vi "celiang.vi"(7 "error in":errorcluster) -> (27 "error out":errorcluster)   [LabVIEW 2014]
uses:
  <vilib>/vision/Image Controls.llb/Vision Info Type2.ctl
  <vilib>/vision/Pattern Matching.llb/IMAQ Curve Parameters.ctl
  <vilib>/vision/NI_Vision_Development_Module.lvlib
panel:
  out "Image Out":T1(plugin-control)
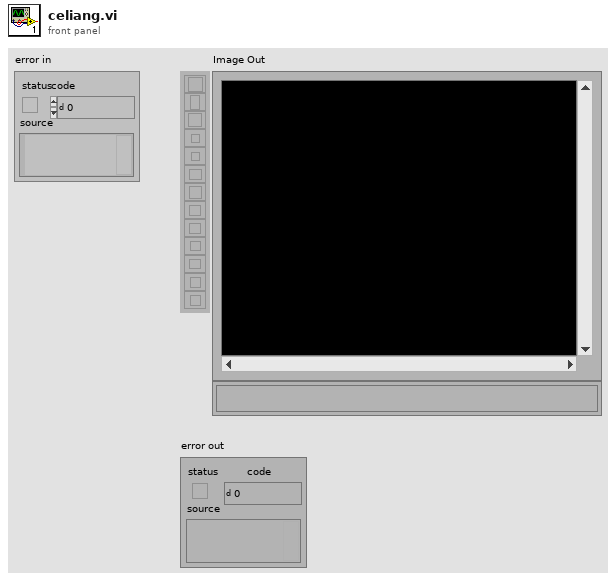
[diagram p1: front panel]
types:
  T1 = typedef "IMAQ Image.ctl" = refnum<image>
  T2 = cluster{"Angle Range (+/-)":dbl, "Edge Polarity":cluster{"Start":u32, "End":u32}}
  T3 = typedef "IMAQ Curve Parameters.ctl" = cluster{"Extraction Mode":u32, "Edge Threshold":i32, "Edge Filter Size":u32, "Min Length":i32, "Row Search Step Size":i32, "Col Search Step Size":i32, "Max Endpoint Gap":i32, "Closed":bool, "Subpixel":bool}
  T4 = cluster{"Show Search Area":bool, "Show Curves":bool, "Show Clamp Locations":bool, "Show Result":bool, "Search Area Color":u32, "Curves Color":u32, "Clamp Locations Color":u32, "Result Color":u32, "Overlay Group Name":string}
  T5 = cluster{"Global Rectangle":i32[], "Contours":cluster{"ID":enum32{"External", "Internal"}, "Type":u32, "Coordinates":i32[]}[]}
  T6 = cluster{"Origin":cluster{"X":sgl, "Y":sgl}, "Angle (deg)":sgl, "Axis Reference":u32}
  T7 = enum16{"Reset", "Update Coordinate System", "Get Coordinate System"}
  T8 = cluster{"Contrast":i32, "Filter width":i32, "Steepness":i32, "Subsampling Ratio":u32, "Show Search Area":bool, "Show Search Lines":bool, "Show Edges Found":bool, "Show Result":bool}
  T9 = enum16{"Horizontal Motion", "Vertical Motion", "Horizontal and Vertical Motion", "Horizontal, Vertical and Angular Motion"}
  T10 = enum16{"Get First Edge", "Get First + Last Edge", "Get All Edges"}
  T11 = cluster{"Level Type":enum32{"Absolute Value", "Relative value"}, "Threshold Level":i32, "Hysteresis":i32}
  T12 = cluster{"Origin Pixel":cluster{"X":sgl, "Y":sgl}, "X Axis Pixel":cluster{"X":sgl, "Y":sgl}, "Axis Reference":u32}
  T13 = typedef "Vision Info Type2.ctl" = u32
  T14 = typedef "Simple Grid Descriptor" = cluster{"X Step":sgl, "Y Step":sgl, "Unit":T15}
  T15 = typedef "Image Unit" = enum32{"Undefined", "Angström", "Micrometer", "Millimeter", "Centimeter", "Meter", "Kilometer", "Microinch", "Inch", "Feet", "Nautical miles", "Standard miles", "Steps"}
  T16 = typedef "Image Type" = u32
  T17 = typedef "IMAQ Coordinate System" = cluster{"Reference System":cluster{"Origin":cluster{"X":sgl, "Y":sgl}, "Angle (deg)":sgl, "Axis Reference":u32}, "Measurement System":cluster{"Origin":cluster{"X":sgl, "Y":sgl}, "Angle (deg)":sgl, "Axis Reference":u32}}
  T18 = typedef "ROI Descriptor" = cluster{"Global Rectangle":i32[], "Contours":cluster{"ID":enum32{"External", "Internal"}, "Type":u32, "Coordinates":i32[]}[]}
  T19 = cluster{"Distance (Pixels)":dbl, "Distance (Real World)":dbl, "Angle (Absolute)":dbl, "Angle (Relative)":dbl}
  T20 = cluster{"Pixels ":cluster{"Start":cluster{"X":dbl, "Y":dbl}, "End":cluster{"X":dbl, "Y":dbl}}, "Real World":cluster{"Start":cluster{"X":dbl, "Y":dbl}, "End":cluster{"X":dbl, "Y":dbl}}}
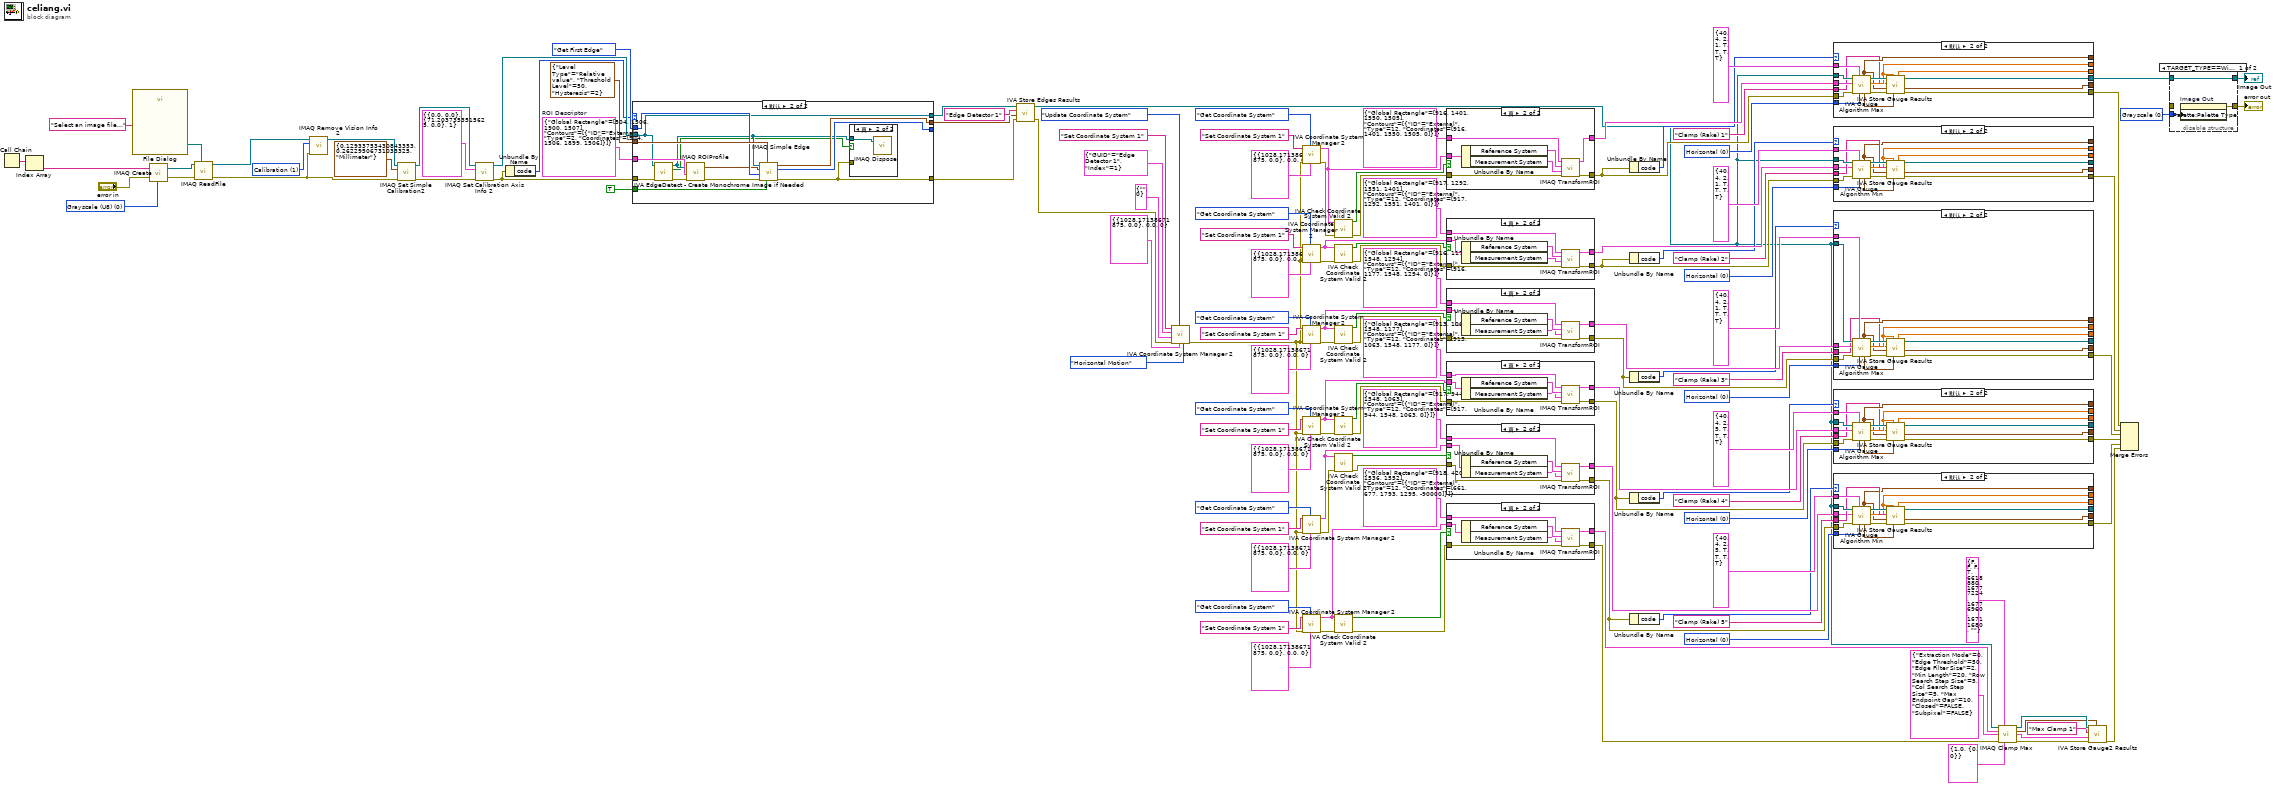
[diagram p0: block diagram]
diagram:
  w1 = u32 0 items=["Grayscale", "Binary", "Gradient", "Rainbow", "Temperature", "User Defined"] ("Palette")
  w33 = u32 0 items=["Horizontal", "Vertical"] ("Scanning axis")
  w49 = u32 0 items=["Horizontal", "Vertical"] ("Scanning axis")
  w63 = u32 0 items=["Horizontal", "Vertical"] ("Scanning axis")
  w75 = u32 0 items=["Horizontal", "Vertical"] ("Scanning axis")
  w91 = u32 0 items=["Horizontal", "Vertical"] ("Scanning axis")
  w112 = T5 {"Global Rectangle"=[504, 1506, 1900, 1507], "Contours"=[{"ID"=enum."External", "Type"=2, "Coordinates"=[504, 1506, 1899, 1506]}]}  # ROI Descriptor
  w125 = T13 1 items=["Any", "Calibration", "Overlay", "Grayscale Template", "Color Template", "Geometric Template", "Custom Data", "Golden Template", "Geometric Template 2", "Contour Data", "Camera Model"] ("Vision Info")
  w127 = T16 0 items=["Grayscale (U8)", "Grayscale (I16)", "Grayscale (SGL)", "Complex (CSG)", "RGB (U32)", "HSL (U32)", "RGB (U64)", "Grayscale (U16)"] ("Image Type")
  n1 = Call Chain() -> (call chain=w131:string[])
  n2 = Index Array(array=w131) -> (element=w130:string)  [unwired: 1 in]
  n3 = call "File Dialog"("prompt"="Select an image file...") -> ("selected path"=w128:path)  [unwired: 6 in, 8 out]
  n4 = call "IMAQ Create"("Image Name"=w130, "Image Type"=w127, "error in (no error)"="error in") -> ("New Image"=w134:T1, "error out"=w133:errorcluster)  [unwired: 1 in, 1 out]
  n5 = call "IMAQ ReadFile"("File Path"=w128, "error in (no error)"=w133, "Image"=w134) -> ("error out"=w122:errorcluster, "Image Out"=w124:T1)  [unwired: 2 in, 5 out]
  n6 = call "IMAQ Remove Vision Info 2"("error in (no error)"=w122, "Vision Info"=w125, "Image"=w124) -> ("Image Out"=w123:T1)  [unwired: 8 out]
  n7 = call "IMAQ Set Simple Calibration2"("error in (no error)"=w122, "Pixel Distances"=T14 {"X Step"=0.12933753, "Y Step"=0.26229507, "Unit"=enum."Millimeter"} ("Grid Descriptor"), "Image"=w123) -> ("error out"=w120:errorcluster, "Calibration Template Image"=w121:T1)  [unwired: 2 in, 5 out]
  n8 = call-poly "IMAQ Set Calibration Axis Info 2"("error in (no error)"=w120, "Calibration Axis Info"=T12 {"Origin Pixel"={"X"=0.0, "Y"=0.0}, "X Axis Pixel"={"X"=71.203735, "Y"=0.0}, "Axis Reference"=1}, "Calibration Template Image In"=w121) -> ("error out"=w111:errorcluster, "Calibration Template Image Out"=w116:T1)  [unwired: 7 out]
  n9 = Unbundle By Name(w111) -> ("code"=w110:i32)
  n10 = case "条件结构" shown="默认" w110 {
    tunnel: T11 {"Level Type"=enum."Relative value", "Threshold Level"=50, "Hysteresis"=2} ("Threshold Parameters") -> [_ w149]
    tunnel: T10."Get First Edge" ("Process") -> [_ w148]
    tunnel: [_ w147] -> _
    tunnel: w111 -> [_ w140]
    tunnel: w116 -> [w135 w141]
    tunnel: [_ w144] -> w114
    tunnel: [_ w136] -> w113
    tunnel: w112 -> [_ w143]
    tunnel: TRUE ("Sub-Pixel Accuracy") -> [_ w142]
    tunnel: [w135 w141] -> w108
    frame -1074396199, -1074396198 {
      # "Discard Coordinate System Error"
    }
    frame Default {
      n11 = call <vilib>:"IVA EdgeDetect - Create Monochrome Image if Needed.vi"("error in (no error)"=w140, "Image In"=w141) -> ("error out"=w139:errorcluster, "Mono Image Created"=w137:bool, "Mono Image Out"=w138:T1)  [unwired: 7 out]
      n12 = call "IMAQ ROIProfile"("error in (no error)"=w139, "ROI Descriptor"=w143, "Image"=w138) -> ("error out"=w145:errorcluster, "Pixel Coordinates"=w146:cluster{"X":u32, "Y":u32}[])  [unwired: 4 out]
      n13 = call "IMAQ Simple Edge"("Sub-Pixel Accuracy"=w142, "Threshold Parameters"=w149, "error in (no error)"=w145, "Process"=w148, "Pixel Coordinates"=w146, "Image Src"=w138) -> ("error out"=w136:errorcluster, "Number of Edges"=w147:i32, "Edges Coordinates"=w144:cluster{"X":sgl, "Y":sgl}[])  [unwired: 3 out]
      n14 = case "条件结构" shown="真" w137 {
        tunnel: w138 -> [_ w150]
        tunnel: w136 -> [_ _]
        frame False {
        }
        frame True {
          n15 = call "IMAQ Dispose"("Image"=w150) -> ()  [unwired: 2 in, 4 out]
        }
      }
    }
  }
  n16 = call <vilib>:"IVA Store Edges Results.vi"("error in (no error)"=w113, "Edge Coordinates"=w114, "Step Name"="Edge Detector 1", "Image in"=w108) -> ("error out"=w101:errorcluster, "Image dup"=w20:T1)  [unwired: 6 out]
  n17 = call <vilib>:"IVA Coordinate System Manager 2.vi"("Mode"=T9."Horizontal Motion", "Reference System"=T6 {"Origin"={"X"=1028.1714, "Y"=0.0}, "Angle (deg)"=0.0, "Axis Reference"=0}, "Function"=T7."Update Coordinate System", "error in (no error)"=w101, "Angle ID"=cluster{"GUID":string, "Index":i32} {"GUID"="", "Index"=0}, "Origin ID"=cluster{"GUID":string, "Index":i32} {"GUID"="Edge Detector 1", "Index"=1}, "Coordinate System Name"="Set Coordinate System 1") -> ("error out"=w28:errorcluster)  [unwired: 4 out]
  n18 = call <vilib>:"IVA Coordinate System Manager 2.vi"("Reference System"=T6 {"Origin"={"X"=1028.1714, "Y"=0.0}, "Angle (deg)"=0.0, "Axis Reference"=0}, "Function"=T7."Get Coordinate System", "error in (no error)"=w28, "Coordinate System Name"="Set Coordinate System 1") -> ("error out"=w94:errorcluster, "Coordinate System Out"=w96:T17)  [unwired: 3 in, 3 out]
  n19 = call <vilib>:"IVA Coordinate System Manager 2.vi"("Reference System"=T6 {"Origin"={"X"=1028.1714, "Y"=0.0}, "Angle (deg)"=0.0, "Axis Reference"=0}, "Function"=T7."Get Coordinate System", "error in (no error)"=w28, "Coordinate System Name"="Set Coordinate System 1") -> ("error out"=w80:errorcluster, "Coordinate System Out"=w82:T17)  [unwired: 3 in, 3 out]
  n20 = call <vilib>:"IVA Coordinate System Manager 2.vi"("Reference System"=T6 {"Origin"={"X"=1028.1714, "Y"=0.0}, "Angle (deg)"=0.0, "Axis Reference"=0}, "Function"=T7."Get Coordinate System", "error in (no error)"=w28, "Coordinate System Name"="Set Coordinate System 1") -> ("error out"=w66:errorcluster, "Coordinate System Out"=w68:T17)  [unwired: 3 in, 3 out]
  n21 = call <vilib>:"IVA Coordinate System Manager 2.vi"("Reference System"=T6 {"Origin"={"X"=1028.1714, "Y"=0.0}, "Angle (deg)"=0.0, "Axis Reference"=0}, "Function"=T7."Get Coordinate System", "error in (no error)"=w28, "Coordinate System Name"="Set Coordinate System 1") -> ("error out"=w52:errorcluster, "Coordinate System Out"=w54:T17)  [unwired: 3 in, 3 out]
  n22 = call <vilib>:"IVA Coordinate System Manager 2.vi"("Reference System"=T6 {"Origin"={"X"=1028.1714, "Y"=0.0}, "Angle (deg)"=0.0, "Axis Reference"=0}, "Function"=T7."Get Coordinate System", "error in (no error)"=w28, "Coordinate System Name"="Set Coordinate System 1") -> ("error out"=w38:errorcluster, "Coordinate System Out"=w40:T17)  [unwired: 3 in, 3 out]
  n23 = call <vilib>:"IVA Coordinate System Manager 2.vi"("Reference System"=T6 {"Origin"={"X"=1028.1714, "Y"=0.0}, "Angle (deg)"=0.0, "Axis Reference"=0}, "Function"=T7."Get Coordinate System", "error in (no error)"=w28, "Coordinate System Name"="Set Coordinate System 1") -> ("error out"=w23:errorcluster, "Coordinate System Out"=w25:T17)  [unwired: 3 in, 3 out]
  n24 = call <vilib>:"IVA Check Coordinate System Valid 2.vi"("error in (no error)"=w94, "Coordinate System"=w96) -> ("error out"=w93:errorcluster, "Valid?"=w95:bool)  [unwired: 8 out]
  n25 = call <vilib>:"IVA Check Coordinate System Valid 2.vi"("error in (no error)"=w80, "Coordinate System"=w82) -> ("error out"=w79:errorcluster, "Valid?"=w81:bool)  [unwired: 8 out]
  n26 = call <vilib>:"IVA Check Coordinate System Valid 2.vi"("error in (no error)"=w66, "Coordinate System"=w68) -> ("error out"=w65:errorcluster, "Valid?"=w67:bool)  [unwired: 8 out]
  n27 = call <vilib>:"IVA Check Coordinate System Valid 2.vi"("error in (no error)"=w52, "Coordinate System"=w54) -> ("error out"=w51:errorcluster, "Valid?"=w53:bool)  [unwired: 8 out]
  n28 = call <vilib>:"IVA Check Coordinate System Valid 2.vi"("error in (no error)"=w38, "Coordinate System"=w40) -> ("error out"=w37:errorcluster, "Valid?"=w39:bool)  [unwired: 8 out]
  n29 = call <vilib>:"IVA Check Coordinate System Valid 2.vi"("error in (no error)"=w23, "Coordinate System"=w25) -> ("error out"=w22:errorcluster, "Valid?"=w24:bool)  [unwired: 8 out]
  n30 = case "条件结构" shown="真" w95 {
    tunnel: T5 {"Global Rectangle"=[916, 1401, 1550, 1505], "Contours"=[{"ID"=enum."External", "Type"=12, "Coordinates"=[916, 1401, 1550, 1505, 0]}]} ("ROI Descriptor") -> [w152 w159]
    tunnel: [w152 w156] -> w90
    tunnel: [w151 w155] -> w89
    tunnel: w96 -> [_ w154]
    tunnel: w93 -> [w151 w153]
    frame False {
    }
    frame True {
      n31 = Unbundle By Name(w154) -> ("Reference System"=w158:T6, "Measurement System"=w157:T6)
      n32 = call "IMAQ TransformROI"("error in (no error)"=w153, "New Reference"=w157, "Base Reference"=w158, "ROI Descriptor"=w159) -> ("error out"=w155:errorcluster, "ROI Descriptor out"=w156:T18)  [unwired: 6 out]
    }
  }
  n33 = case "条件结构" shown="真" w81 {
    tunnel: T5 {"Global Rectangle"=[917, 1292, 1551, 1401], "Contours"=[{"ID"=enum."External", "Type"=12, "Coordinates"=[917, 1292, 1551, 1401, 0]}]} ("ROI Descriptor") -> [w161 w168]
    tunnel: [w161 w165] -> w76
    tunnel: [w160 w164] -> w74
    tunnel: w82 -> [_ w163]
    tunnel: w79 -> [w160 w162]
    frame False {
    }
    frame True {
      n34 = Unbundle By Name(w163) -> ("Reference System"=w167:T6, "Measurement System"=w166:T6)
      n35 = call "IMAQ TransformROI"("error in (no error)"=w162, "New Reference"=w166, "Base Reference"=w167, "ROI Descriptor"=w168) -> ("error out"=w164:errorcluster, "ROI Descriptor out"=w165:T18)  [unwired: 6 out]
    }
  }
  n36 = case "条件结构" shown="真" w67 {
    tunnel: T5 {"Global Rectangle"=[916, 1177, 1548, 1294], "Contours"=[{"ID"=enum."External", "Type"=12, "Coordinates"=[916, 1177, 1548, 1294, 0]}]} ("ROI Descriptor") -> [w170 w177]
    tunnel: [w170 w174] -> w62
    tunnel: [w169 w173] -> w61
    tunnel: w68 -> [_ w172]
    tunnel: w65 -> [w169 w171]
    frame False {
    }
    frame True {
      n37 = Unbundle By Name(w172) -> ("Reference System"=w176:T6, "Measurement System"=w175:T6)
      n38 = call "IMAQ TransformROI"("error in (no error)"=w171, "New Reference"=w175, "Base Reference"=w176, "ROI Descriptor"=w177) -> ("error out"=w173:errorcluster, "ROI Descriptor out"=w174:T18)  [unwired: 6 out]
    }
  }
  n39 = case "条件结构" shown="真" w53 {
    tunnel: T5 {"Global Rectangle"=[913, 1063, 1548, 1177], "Contours"=[{"ID"=enum."External", "Type"=12, "Coordinates"=[913, 1063, 1548, 1177, 0]}]} ("ROI Descriptor") -> [w179 w186]
    tunnel: [w179 w183] -> w48
    tunnel: [w178 w182] -> w47
    tunnel: w54 -> [_ w181]
    tunnel: w51 -> [w178 w180]
    frame False {
    }
    frame True {
      n40 = Unbundle By Name(w181) -> ("Reference System"=w185:T6, "Measurement System"=w184:T6)
      n41 = call "IMAQ TransformROI"("error in (no error)"=w180, "New Reference"=w184, "Base Reference"=w185, "ROI Descriptor"=w186) -> ("error out"=w182:errorcluster, "ROI Descriptor out"=w183:T18)  [unwired: 6 out]
    }
  }
  n42 = case "条件结构" shown="真" w39 {
    tunnel: T5 {"Global Rectangle"=[917, 944, 1548, 1063], "Contours"=[{"ID"=enum."External", "Type"=12, "Coordinates"=[917, 944, 1548, 1063, 0]}]} ("ROI Descriptor") -> [w188 w195]
    tunnel: [w188 w192] -> w34
    tunnel: [w187 w191] -> w32
    tunnel: w40 -> [_ w190]
    tunnel: w37 -> [w187 w189]
    frame False {
    }
    frame True {
      n43 = Unbundle By Name(w190) -> ("Reference System"=w194:T6, "Measurement System"=w193:T6)
      n44 = call "IMAQ TransformROI"("error in (no error)"=w189, "New Reference"=w193, "Base Reference"=w194, "ROI Descriptor"=w195) -> ("error out"=w191:errorcluster, "ROI Descriptor out"=w192:T18)  [unwired: 6 out]
    }
  }
  n45 = case "条件结构" shown="真" w24 {
    tunnel: T5 {"Global Rectangle"=[918, 420, 1536, 1552], "Contours"=[{"ID"=enum."External", "Type"=12, "Coordinates"=[661, 677, 1793, 1295, -90000]}]} ("ROI Descriptor") -> [w197 w204]
    tunnel: [w197 w201] -> w15
    tunnel: [w196 w200] -> w19
    tunnel: w25 -> [_ w199]
    tunnel: w22 -> [w196 w198]
    frame False {
    }
    frame True {
      n46 = Unbundle By Name(w199) -> ("Reference System"=w203:T6, "Measurement System"=w202:T6)
      n47 = call "IMAQ TransformROI"("error in (no error)"=w198, "New Reference"=w202, "Base Reference"=w203, "ROI Descriptor"=w204) -> ("error out"=w200:errorcluster, "ROI Descriptor out"=w201:T18)  [unwired: 6 out]
    }
  }
  n48 = Unbundle By Name(w89) -> ("code"=w88:i32)
  n49 = Unbundle By Name(w74) -> ("code"=w73:i32)
  n50 = Unbundle By Name(w61) -> ("code"=w60:i32)
  n51 = Unbundle By Name(w47) -> ("code"=w46:i32)
  n52 = Unbundle By Name(w32) -> ("code"=w31:i32)
  n53 = case "条件结构" shown="默认" w88 {
    tunnel: w20 -> [w205 w220]
    tunnel: w89 -> [_ w219]
    tunnel: T8 {"Contrast"=40, "Filter width"=4, "Steepness"=2, "Subsampling Ratio"=1, "Show Search Area"=TRUE, "Show Search Lines"=TRUE, "Show Edges Found"=TRUE, "Show Result"=TRUE} ("Settings") -> [_ w218]
    tunnel: w91 -> [_ w217]
    tunnel: w90 -> [_ w216]
    tunnel: [w205 w214] -> w3
    tunnel: [_ w212] -> w10
    tunnel: [_ w211] -> _
    tunnel: [_ w210] -> _
    tunnel: [_ w209] -> _
    tunnel: [_ w208] -> _
    tunnel: "Clamp (Rake) 1" ("Step Name") -> [_ w207]
    frame -1074396199, -1074396198 {
      # "Discard Coordinate System Error"
    }
    frame Default {
      n54 = call <vilib>:"IVA Gauge Algorithm Max.vi"("Scanning axis"=w217, "Settings"=w218, "error in (no error)"=w219, "ROI Descriptor"=w216, "Image"=w220) -> ("error out"=w213:errorcluster, "Distance"=w211:sgl, "Image Out"=w215:T1, "Distance Points"=w206:cluster{"X":sgl, "Y":sgl}[], "Points of Contact"=w210:cluster{"X":sgl, "Y":sgl}[])  [unwired: 1 in, 1 out]
      n55 = call <vilib>:"IVA Store Gauge Results.vi"("Distance Points"=w206, "Distance"=w211, "error in (no error)"=w213, "Points of Contact"=w210, "Step Name"=w207, "Image in"=w215) -> ("error out"=w212:errorcluster, "Points of Contact (calibrated)"=w208:cluster{"X":sgl, "Y":sgl}[], "Image dup"=w214:T1, "Distance (calibrated)"=w209:sgl)  [unwired: 2 out]
    }
  }
  n56 = case "条件结构" shown="默认" w73 {
    tunnel: T8 {"Contrast"=40, "Filter width"=4, "Steepness"=2, "Subsampling Ratio"=1, "Show Search Area"=TRUE, "Show Search Lines"=TRUE, "Show Edges Found"=TRUE, "Show Result"=TRUE} ("Settings") -> [_ w236]
    tunnel: w20 -> [w221 w235]
    tunnel: w74 -> [_ w234]
    tunnel: [w221 w232] -> _
    tunnel: [_ w230] -> w9
    tunnel: "Clamp (Rake) 2" ("Step Name") -> [_ w229]
    tunnel: [_ w228] -> _
    tunnel: [_ w226] -> _
    tunnel: [_ w225] -> _
    tunnel: w76 -> [_ w224]
    tunnel: w75 -> [_ w223]
    tunnel: [_ w222] -> _
    frame -1074396199, -1074396198 {
      # "Discard Coordinate System Error"
    }
    frame Default {
      n57 = call <vilib>:"IVA Gauge Algorithm Min.vi"("Scanning axis"=w223, "Settings"=w236, "error in (no error)"=w234, "ROI Descriptor"=w224, "Image"=w235) -> ("error out"=w231:errorcluster, "Distance"=w228:sgl, "Image Out"=w233:T1, "Distance Points"=w227:cluster{"X":sgl, "Y":sgl}[], "Edge Coordinates"=w226:cluster{"X":sgl, "Y":sgl}[])  [unwired: 1 in, 1 out]
      n58 = call <vilib>:"IVA Store Gauge Results.vi"("Distance Points"=w227, "Distance"=w228, "error in (no error)"=w231, "Points of Contact"=w226, "Step Name"=w229, "Image in"=w233) -> ("error out"=w230:errorcluster, "Points of Contact (calibrated)"=w222:cluster{"X":sgl, "Y":sgl}[], "Image dup"=w232:T1, "Distance (calibrated)"=w225:sgl)  [unwired: 2 out]
    }
  }
  n59 = case "条件结构" shown="默认" w60 {
    tunnel: w20 -> [w237 w252]
    tunnel: w61 -> [_ w251]
    tunnel: T8 {"Contrast"=40, "Filter width"=4, "Steepness"=2, "Subsampling Ratio"=1, "Show Search Area"=TRUE, "Show Search Lines"=TRUE, "Show Edges Found"=TRUE, "Show Result"=TRUE} ("Settings") -> [_ w250]
    tunnel: w63 -> [_ w249]
    tunnel: w62 -> [_ w248]
    tunnel: [w237 w246] -> _
    tunnel: [_ w244] -> w8
    tunnel: [_ w243] -> _
    tunnel: [_ w242] -> _
    tunnel: [_ w241] -> _
    tunnel: [_ w240] -> _
    tunnel: "Clamp (Rake) 3" ("Step Name") -> [_ w239]
    frame -1074396199, -1074396198 {
      # "Discard Coordinate System Error"
    }
    frame Default {
      n60 = call <vilib>:"IVA Gauge Algorithm Max.vi"("Scanning axis"=w249, "Settings"=w250, "error in (no error)"=w251, "ROI Descriptor"=w248, "Image"=w252) -> ("error out"=w245:errorcluster, "Distance"=w243:sgl, "Image Out"=w247:T1, "Distance Points"=w238:cluster{"X":sgl, "Y":sgl}[], "Points of Contact"=w242:cluster{"X":sgl, "Y":sgl}[])  [unwired: 1 in, 1 out]
      n61 = call <vilib>:"IVA Store Gauge Results.vi"("Distance Points"=w238, "Distance"=w243, "error in (no error)"=w245, "Points of Contact"=w242, "Step Name"=w239, "Image in"=w247) -> ("error out"=w244:errorcluster, "Points of Contact (calibrated)"=w240:cluster{"X":sgl, "Y":sgl}[], "Image dup"=w246:T1, "Distance (calibrated)"=w241:sgl)  [unwired: 2 out]
    }
  }
  n62 = case "条件结构" shown="默认" w46 {
    tunnel: w20 -> [w253 w268]
    tunnel: w47 -> [_ w267]
    tunnel: T8 {"Contrast"=40, "Filter width"=4, "Steepness"=2, "Subsampling Ratio"=5, "Show Search Area"=TRUE, "Show Search Lines"=TRUE, "Show Edges Found"=TRUE, "Show Result"=TRUE} ("Settings") -> [_ w266]
    tunnel: w49 -> [_ w265]
    tunnel: w48 -> [_ w264]
    tunnel: [w253 w262] -> _
    tunnel: [_ w260] -> w7
    tunnel: [_ w259] -> _
    tunnel: [_ w258] -> _
    tunnel: [_ w257] -> _
    tunnel: [_ w256] -> _
    tunnel: "Clamp (Rake) 4" ("Step Name") -> [_ w255]
    frame -1074396199, -1074396198 {
      # "Discard Coordinate System Error"
    }
    frame Default {
      n63 = call <vilib>:"IVA Gauge Algorithm Max.vi"("Scanning axis"=w265, "Settings"=w266, "error in (no error)"=w267, "ROI Descriptor"=w264, "Image"=w268) -> ("error out"=w261:errorcluster, "Distance"=w259:sgl, "Image Out"=w263:T1, "Distance Points"=w254:cluster{"X":sgl, "Y":sgl}[], "Points of Contact"=w258:cluster{"X":sgl, "Y":sgl}[])  [unwired: 1 in, 1 out]
      n64 = call <vilib>:"IVA Store Gauge Results.vi"("Distance Points"=w254, "Distance"=w259, "error in (no error)"=w261, "Points of Contact"=w258, "Step Name"=w255, "Image in"=w263) -> ("error out"=w260:errorcluster, "Points of Contact (calibrated)"=w256:cluster{"X":sgl, "Y":sgl}[], "Image dup"=w262:T1, "Distance (calibrated)"=w257:sgl)  [unwired: 2 out]
    }
  }
  n65 = case "条件结构" shown="默认" w31 {
    tunnel: T8 {"Contrast"=40, "Filter width"=4, "Steepness"=2, "Subsampling Ratio"=5, "Show Search Area"=TRUE, "Show Search Lines"=TRUE, "Show Edges Found"=TRUE, "Show Result"=TRUE} ("Settings") -> [_ w284]
    tunnel: w20 -> [w269 w283]
    tunnel: w32 -> [_ w282]
    tunnel: [w269 w280] -> _
    tunnel: [_ w278] -> w6
    tunnel: "Clamp (Rake) 5" ("Step Name") -> [_ w277]
    tunnel: [_ w276] -> _
    tunnel: [_ w274] -> _
    tunnel: [_ w273] -> _
    tunnel: w34 -> [_ w272]
    tunnel: w33 -> [_ w271]
    tunnel: [_ w270] -> _
    frame -1074396199, -1074396198 {
      # "Discard Coordinate System Error"
    }
    frame Default {
      n66 = call <vilib>:"IVA Gauge Algorithm Min.vi"("Scanning axis"=w271, "Settings"=w284, "error in (no error)"=w282, "ROI Descriptor"=w272, "Image"=w283) -> ("error out"=w279:errorcluster, "Distance"=w276:sgl, "Image Out"=w281:T1, "Distance Points"=w275:cluster{"X":sgl, "Y":sgl}[], "Edge Coordinates"=w274:cluster{"X":sgl, "Y":sgl}[])  [unwired: 1 in, 1 out]
      n67 = call <vilib>:"IVA Store Gauge Results.vi"("Distance Points"=w275, "Distance"=w276, "error in (no error)"=w279, "Points of Contact"=w274, "Step Name"=w277, "Image in"=w281) -> ("error out"=w278:errorcluster, "Points of Contact (calibrated)"=w270:cluster{"X":sgl, "Y":sgl}[], "Image dup"=w280:T1, "Distance (calibrated)"=w273:sgl)  [unwired: 2 out]
    }
  }
  n68 = call "IMAQ Clamp Max"("Source Image"=w20, "Overlay Settings"=T4 {"Show Search Area"=FALSE, "Show Curves"=FALSE, "Show Clamp Locations"=FALSE, "Show Result"=TRUE, "Search Area Color"=6618880, "Curves Color"=16777224, "Clamp Locations Color"=16776960, "Result Color"=16711680, "Overlay Group Name"=""}, "ROI Descriptor"=w15, "Curve Extraction Settings"=T3 {"Extraction Mode"=0, "Edge Threshold"=50, "Edge Filter Size"=2, "Min Length"=20, "Row Search Step Size"=5, "Col Search Step Size"=5, "Max Endpoint Gap"=10, "Closed"=FALSE, "Subpixel"=FALSE}, "error in (no error)"=w19, "Clamp Settings"=T2 {"Angle Range (+/-)"=1.0, "Edge Polarity"={"Start"=0, "End"=0}}) -> ("Image Out"=w18:T1, "Clamp Results"=w12:T19, "Clamp Points"=w11:T20, "error out"=w21:errorcluster)  [unwired: 1 in, 5 out]
  n69 = call <vilib>:"IVA Store Gauge2 Results.vi"("Clamp Results"=w12, "error in (no error)"=w21, "Clamp Points"=w11, "Step Name"="Max Clamp 1", "Image in"=w18) -> ("error out"=w5:errorcluster)  [unwired: 6 out]
  n70 = Merge Errors(w10, w9, w8, w7, w6, w5) -> ()  [unwired: 1 out]
  n71 = disable-structure "条件禁用结构" shown="TARGET_TYPE==Windows" {
    disable-tunnel: _ -> [_ w288]
    disable-tunnel: [w287 w288] -> w4
    disable-tunnel: w3 -> [w286 w289]
    disable-tunnel: [w286 w289] -> w2
    disable-tunnel: w1 -> [w285 _]
    frame condition #0 (active) {
      n72 = property on="Image Out" class="ImageControl"("Palette:Palette Type"=w285) -> (error out=w287:errorcluster)  [unwired: 2 in, 1 out]
    }
    frame condition #1 {
    }
  }
  "error out" <- w4
  "Image Out" <- w2
